vi "Read ChnParameter.vi"(8 "error in (no error)":errorcluster, 11 "BME_DG_Chnl in":refnum<class "BME_DG_Chnl.lvclass">) -> (0 "error out":errorcluster, 1 "Nr":i32, 2 "ChnParemater":T1 {"Delay (µs)" min=0.0 max=100000000.0 format="%.5f"}, 3 "BME_DG_Chnl out":refnum<class "BME_DG_Chnl.lvclass">, 4 "DG Nr":i32, 5 "Name":string)   [LabVIEW 2009, in "POLARIS BME DG.lvlib" / "BME_DG_Chnl.lvclass"]
uses:
  BME_DG_Chnl.lvclass
  LV-BME Interface/ChnlSettings.ctl
  BME_DG_Chnl.lvclass/BME_DG_Chnl.ctl
  POLARIS BME DG.lvlib
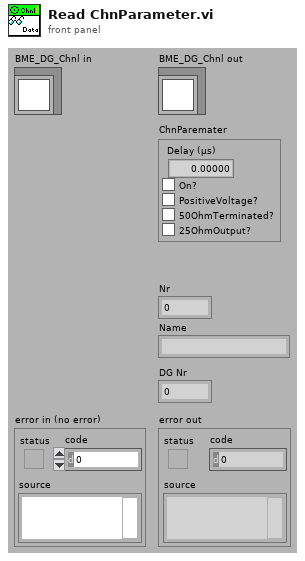
[diagram p1: front panel]
types:
  T1 = typedef "POLARIS BME DG.lvlib/ChnlSettings.ctl" = cluster{" Delay (µs)":dbl, "On?":bool, "PositiveVoltage?":bool, "50OhmTerminated? ":bool, "25OhmOutput?":bool}
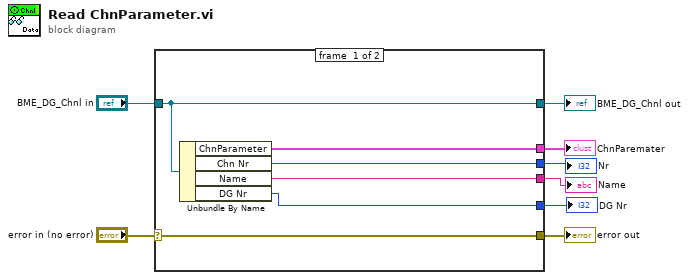
[diagram p0: block diagram]
diagram:
  n1 = case shown="No Error" "error in (no error)" {
    selector: "error in (no error)" -> [w14 w15]
    tunnel: [w14 w15] -> w7
    tunnel: [w13 w16] -> w5
    tunnel: "BME_DG_Chnl in" -> [w13 w16]
    tunnel: [w12 _] -> w4
    tunnel: [w11 _] -> w3
    tunnel: [w10 _] -> w2
    tunnel: [w9 _] -> w1
    frame #0 {
      n2 = Unbundle By Name(w13) -> ("ChnParameter"=w12:T1, "Chn Nr"=w11:i32, "Name"=w10:string, "DG Nr"=w9:i32)
    }
    frame #1 {
    }
  }
  "error out" <- w7
  "BME_DG_Chnl out" <- w5
  "ChnParemater" <- w4
  "Nr" <- w3
  "Name" <- w2
  "DG Nr" <- w1
